vi "drive_forward.vi"(8 "min distance":i32=50, 9 "power":i32=50, 11 "NXT":T1) -> (0 "stuck":bool, 3 "NXT 2":T1 caption="NXT")   [LabVIEW 2012]
uses:
  <vilib>/NXT/Subs/LVHSConnector.ctl
  <vilib>/NXT/Subs/MotorOutput.ctl
  <vilib>/NXT/Block Support/NXT_InputPort.ctl
  <vilib>/NXT/Dual Mode Library/Motors/MotorReverse.vi
  <vilib>/NXT/Dual Mode Library/Waits/Wait_Num(msec).vi
  <vilib>/NXT/Dual Mode Library/Motors/MotorBrake.vi
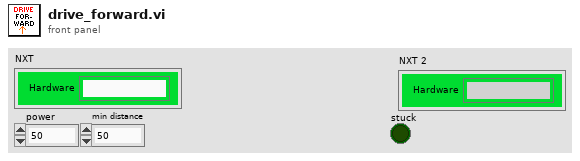
[diagram p1: front panel]
types:
  T1 = typedef "LVHSConnector.ctl" = cluster{"Hardware":string, "Flattened String":string}
  T2 = typedef "MotorOutput.ctl" = u8
  T3 = typedef "NXT_InputPort.ctl" = u8
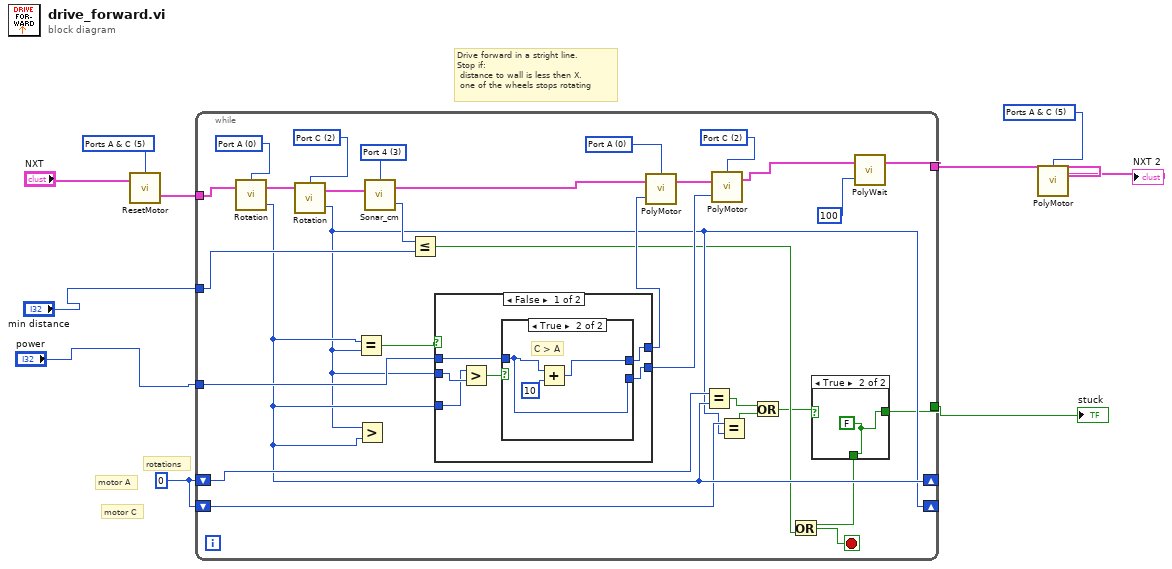
[diagram p0: block diagram]
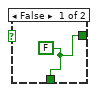
[diagram p2: hidden frame]
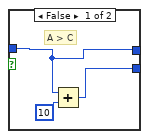
[diagram p3: hidden frame]
diagram:
  w7 = 0
  w10 = T2 5 items=["Port A"=0, "Port B"=1, "Port C"=2, "Ports A & B"=4, "Ports A & C"=5, "Ports B & C"=6, "All Ports"=3] ("Output Port (All Ports)")
  w8 = T2 5 items=["Port A"=0, "Port B"=1, "Port C"=2, "Ports A & B"=4, "Ports A & C"=5, "Ports B & C"=6, "All Ports"=3] ("Output Port (All Ports)")
  # "Drive forward in a stright line.\nStop if:\n distance to wall is less then X.\n one of the wheels stops rotating"
  # "rotations"
  # "motor C"
  # "motor A"
  n1 = call <vilib>:"ResetMotor.vi"("NXT"="NXT", "Port (All Ports)"=w8) -> ("NXT"=w9:T1)  [unwired: 2 in]
  n2 = while {
    tunnel: w9 -> [w39]
    tunnel: [w26] -> w6
    shift-right: [w20] -> _
    shift-left: w7 -> [w21]
    shift-right: [w16] -> _
    shift-left: w7 -> [w17]
    tunnel: "min distance" -> [w28]
    tunnel: "power" -> [w24]
    tunnel: [w11] -> w1
    stop <- w14 stop-if-true
    w32 = T2 2 items=["Port A"=0, "Port B"=1, "Port C"=2, "Ports A & B"=4, "Ports A & C"=5, "Ports B & C"=6, "All Ports"=3] ("Output Port (All Ports)")
    w33 = T2 0 items=["Port A"=0, "Port B"=1, "Port C"=2, "Ports A & B"=4, "Ports A & C"=5, "Ports B & C"=6, "All Ports"=3] ("Output Port (All Ports)")
    w34 = T2 2 items=["Port A"=0, "Port B"=1, "Port C"=2, "Ports A & B"=4, "Ports A & C"=5, "Ports B & C"=6, "All Ports"=3] ("Output Port (All Ports)")
    w35 = T2 0 items=["Port A"=0, "Port B"=1, "Port C"=2, "Ports A & B"=4, "Ports A & C"=5, "Ports B & C"=6, "All Ports"=3] ("Output Port (All Ports)")
    w40 = T3 3 items=["Port 1", "Port 2", "Port 3", "Port 4"] ("Port (Port 4)")
    n3 = call <vilib>:"Rotation.vi"("NXT"=w39, "Port (Port A)"=w33) -> ("Angle of Rotation"=w20:i32, "NXT"=w38:T1)  [unwired: 1 in]
    n4 = call <vilib>:"Rotation.vi"("NXT"=w38, "Port (Port A)"=w32) -> ("Angle of Rotation"=w16:i32, "NXT"=w37:T1)  [unwired: 1 in]
    n5 = Equal?(x=w20, y=w16) -> (x = y?=w31:bool)
    n6 = Greater?(x=w16, y=w20) -> ()  [unwired: 1 out]
    n7 = call <vilib>:"Sonar_cm.vi"("NXT"=w37, "Port (Port 4)"=w40) -> ("Distance (cm)"=w29:i16, "NXT"=w30:T1)  [unwired: 1 in]
    n8 = Less Or Equal?(x=w29, y=w28) -> (x <= y?=w15:bool)
    n9 = case shown="False" w31 {
      tunnel: [w46 w55] -> w27
      tunnel: w24 -> [w47 w55]
      tunnel: [w45 w55] -> w23
      tunnel: w16 -> [w44 _]
      tunnel: w20 -> [w43 _]
      frame False {
        n10 = Greater?(x=w43, y=w44) -> (0:w48:bool)
        n11 = case shown="True" w48 {
          tunnel: w47 -> [w49 w52]
          tunnel: [w49 w53] -> w46
          tunnel: [w50 w52] -> w45
          frame False {
            # "A > C"
            n12 = Add(x=w49, y=10) -> (x+y=w50:i32)
          }
          frame True {
            # "C > A"
            n13 = Add(x=w52, y=10) -> (x+y=w53:i32)
          }
        }
      }
      frame True {
      }
    }
    n14 = call-poly <vilib>:"PolyMotor.vi"("Power (75)"=w27, "NXT"=w30, "Output Port (All Ports)"=w35) -> ("NXT"=w36:T1)  [unwired: 1 in]
    n15 = Equal?(x=w21, y=w20) -> (x = y?=w19:bool)
    n16 = call-poly <vilib>:"PolyMotor.vi"("Power (75)"=w23, "NXT"=w36, "Output Port (All Ports)"=w34) -> ("NXT"=w22:T1)  [unwired: 1 in]
    n17 = Equal?(x=w17, y=w16) -> (x = y?=w18:bool)
    n18 = Or(x=w19, y=w18) -> (x .or. y?=w13:bool)
    n19 = case shown="True" w13 {
      tunnel: [w41 w42] -> w12
      tunnel: [w41 w42] -> w11
      frame False {
        w41 = FALSE
      }
      frame True {
        w42 = FALSE
      }
    }
    n20 = Or(x=w12, y=w15) -> (x .or. y?=w14:bool)
    n21 = call-poly <vilib>:"PolyWait.vi"("Time (100 msec)"=100, "NXT"=w22) -> ("NXT"=w26:T1)  [unwired: 2 in]
  }
  "stuck" <- w1
  n22 = call-poly <vilib>:"PolyMotor.vi"("NXT"=w6, "Port (All Ports)"=w10) -> ("NXT"=→"NXT 2":T1)  [unwired: 2 in]
